vi "SVPO Integration (N CH DBL Array).vi"(6 "reset filters":bool, 9 "highpass cutoff frequency [Hz]":dbl=1.0 format="%.2f", 10 "sampling rate [Hz]":dbl=1.0, 11 "scaled signals [EU]":dbl[][](array[numeric])) -> (3 "integrated signals [EU*s]":dbl[][](array[numeric]))   [LabVIEW 2017, in "SoundVib_Integration.lvlib"]
doc: "Converts acceleration to velocity or velocity to displacement using a time-domain waveform as the input. Wire data to the <B>scaled signal [EU]</B> input to determine the polymorphic instance to use or manually select the instance. This VI performs Single Integration only. You can pass the integrated signal [EU*s] output to the scaled signal [EU] input of second call to this VI to perform double integration."
uses:
  <vilib>/addons/Sound and Vibration/svt_Integration/SoundVib_Integration.lvlib
  <vilib>/addons/_NISVFA/_Shared subVIs/Controls/svc_Integration State.ctl
  <vilib>/addons/Sound and Vibration/svt_Integration/subVIs/svl_Apply Highpass Filter with IC.vi
  <vilib>/addons/Sound and Vibration/svt_Integration/subVIs/svl_Low Pass [Order 1] No State.vi
  <vilib>/addons/Sound and Vibration/svt_Integration/subVIs/svl_Design HighPass Filter.vi
  <vilib>/addons/Sound and Vibration/svt_Integration/subVIs/svl_RC Filter Coefficients.vi
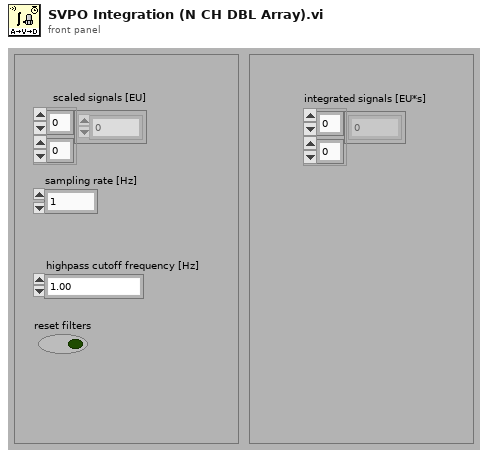
[diagram p1: front panel]
types:
  T1 = typedef "svc_Integration State.ctl" = cluster{"filter coefficents":cluster{"integration filter coefficients":cluster{"beta":dbl, "gamma":dbl, "alpha":dbl}, "highpass filter coefficients":cluster{"filter structure":enum32{"IIR 2nd Order", "IIR 4th Order"}, "Reverse Coefficients":dbl[], "Forward Coefficients":dbl[]}}, "filter state":cluster{"initial integration fiter state":cluster{"x(n-1) state":dbl, "y(n-1) state":dbl, "x(n-2) state":dbl, "y(n-2) state":dbl}, "initial highpass filter state":dbl[]}}
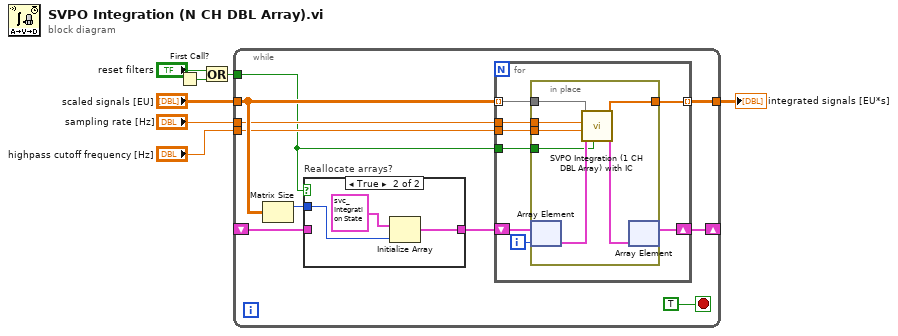
[diagram p0: block diagram]
diagram:
  n1 = First Call?() -> (First Call?: T/F=w7:bool)
  n2 = Or(x="reset filters", y=w7) -> (x .or. y?=w2:bool)
  n3 = while {
    tunnel: "sampling rate [Hz]" -> [w12]
    tunnel: "highpass cutoff frequency [Hz]" -> [w11]
    tunnel: "scaled signals [EU]" -> [w15]
    tunnel: w2 -> [w8]
    tunnel: [w16] -> w1
    shift-right: [w10] -> _
    shift-left: _ -> [w9]
    stop <- TRUE stop-if-true
    n4 = Matrix Size(0:w15) -> (1:w17:i32)  [unwired: 1 out]
    n5 = case "Reallocate arrays?" shown="True" w8 {
      tunnel: [w33 w36] -> w14
      tunnel: w17 -> [_ w34]
      tunnel: w9 -> [w33 _]
      frame False {
      }
      frame True {
        n6 = Initialize Array(T1 {"filter coefficents"={"integration filter coefficients"={"beta"=0.0, "gamma"=0.0, "alpha"=0.0}, "highpass filter coefficients"={"filter structure"=enum."IIR 2nd Order", "Reverse Coefficients"=[], "Forward Coefficients"=[]}}, "filter state"={"initial integration fiter state"={"x(n-1) state"=0.0, "y(n-1) state"=0.0, "x(n-2) state"=0.0, "y(n-2) state"=0.0}, "initial highpass filter state"=[]}} ("Final Conditions"), w34) -> (w36:T1[])
      }
    }
    n7 = for {
      tunnel: [w24] -> w16 mode=indexing
      tunnel: w15 -> [w25] mode=indexing
      tunnel: w12 -> [w21]
      tunnel: w11 -> [w20]
      tunnel: w8 -> [w18]
      shift-right: [w19] -> w10
      shift-left: w14 -> [w22]
      i -> [w23]
      n8 = in-place {
        in-place-border: w25 -> [w32]
        in-place-border: [w31] -> w24
        in-place-border: w21 -> [w28]
        in-place-border: w20 -> [w27]
        in-place-border: w18 -> [w26]
        n9 = in-place-array #1(w22, w23) -> (w30:T1)
        n10 = call <vilib>:"SVPO Integration (1 CH DBL Array) with IC.vi"("reset filters"=w26, "initial conditions"=w30, "highpass cutoff frequency [Hz]"=w27, "sampling rate [Hz]"=w28, "scaled signal [EU]"=w32) -> ("final conditions"=w29:T1, "integrated signal [EU*s]"=w31:dbl[])  [unwired: 5 in]
        n11 = in-place-array #1(w29) -> (w19:T1[])  [unwired: 1 out]
      }
    }
  }
  "integrated signals [EU*s]" <- w1
